vi "GetClassLibFromIDNStr.vi"(8 "error in":errorcluster, 10 "IDNStr":string, 11 "Driver folder":path) -> (0 "error out":errorcluster, 3 "object":refnum<class>)   [LabVIEW 2014]
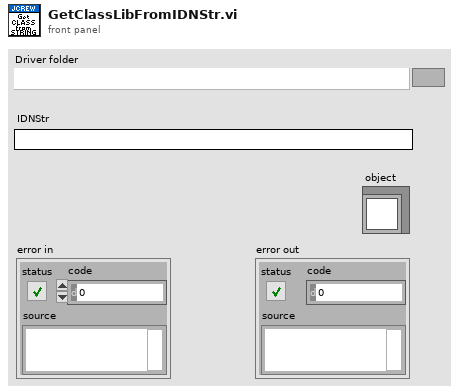
[diagram p1: front panel]
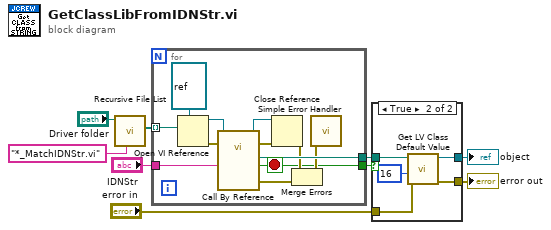
[diagram p0: block diagram]
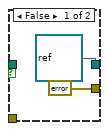
[diagram p2: hidden frame]
diagram:
  n1 = call <vilib>:"Recursive File List.vi"("pattern"="*_MatchIDNStr.vi", "Folder Path"="Driver folder") -> ("All Files in Dir"=w7:path[])  [unwired: 5 in, 4 out]
  n2 = for {
    tunnel: w7 -> [w18] mode=indexing
    tunnel: "IDNStr" -> [w17]
    tunnel: [w16] -> w5
    tunnel: [w10] -> w1
    stop <- w10 stop-if-true
    n3 = Open VI Reference(type specifier VI Refnum (for type only)=refnum<vi> refnum, vi path=w18) -> (vi reference=w20:refnum<vi>, error out=w15:errorcluster)  [unwired: 4 in]
    n4 = call-by-ref "?"(reference=w20, error in=w15, "IDNStr"=w17) -> (reference out=w19:refnum<vi>, error out=w14:errorcluster, 0:"error out"=w13:errorcluster, "IDN match"=w10:bool, "ClassLibraryFile"=w16:path)  [unwired: 8 in]
    n5 = Close Reference(reference=w19, error in (no error)=w14) -> (error out=w12:errorcluster)
    n6 = Merge Errors(w12, w13) -> (w11:errorcluster)
    n7 = call <vilib>:"Simple Error Handler.vi"("error in (no error)"=w11) -> ()  [unwired: 4 in, 5 out]
  }
  n8 = case shown="True" w1 {
    tunnel: w5 -> [_ w28]
    tunnel: "error in" -> [_ w27]
    tunnel: [refnum<class> refnum ("object") w26] -> w3
    tunnel: [errorcluster {"status"=TRUE, "code"=-23456, "source"="Failed to match IDN string to any Instrument class"} ("error out") w25] -> w2
    frame False {
    }
    frame True {
      n9 = call <vilib>:"Get LV Class Default Value.vi"("error in (no error)"=w27, "options"=u32 16, "class path"=w28) -> ("error out"=w25:errorcluster, "object"=w26:refnum<class>)  [unwired: 7 in]
    }
  }
  "error out" <- w2
  "object" <- w3
